vi "Auto.vi"() -> ()   [LabVIEW 2018]
uses:
  Controls/READ CAN CLUSTER.ctl
  CAN_States.ctl
  Controls/FEV_DBC CLUSTER.ctl
  Controls/DBC CLUSTER.ctl
  Controls/CLUSTER.ctl
  CAN Write Data/Application/Common VIs/Read File Data.ctl
  Conf/FGV States.ctl
  cc4f6fa3-47e0-4703-a92c-c7cffe72e988.vi
panel:
  in  "SEND DATA":bool
  in  "TRIGGER":bool
  in  "READ DATA":bool
  in  "exit":bool
  in  "error in (no error)":errorcluster
  out "error out":errorcluster
  in  "WRITE DATA":T1[](array[typedef])
  out "READ DATA":T1[](array[typedef])
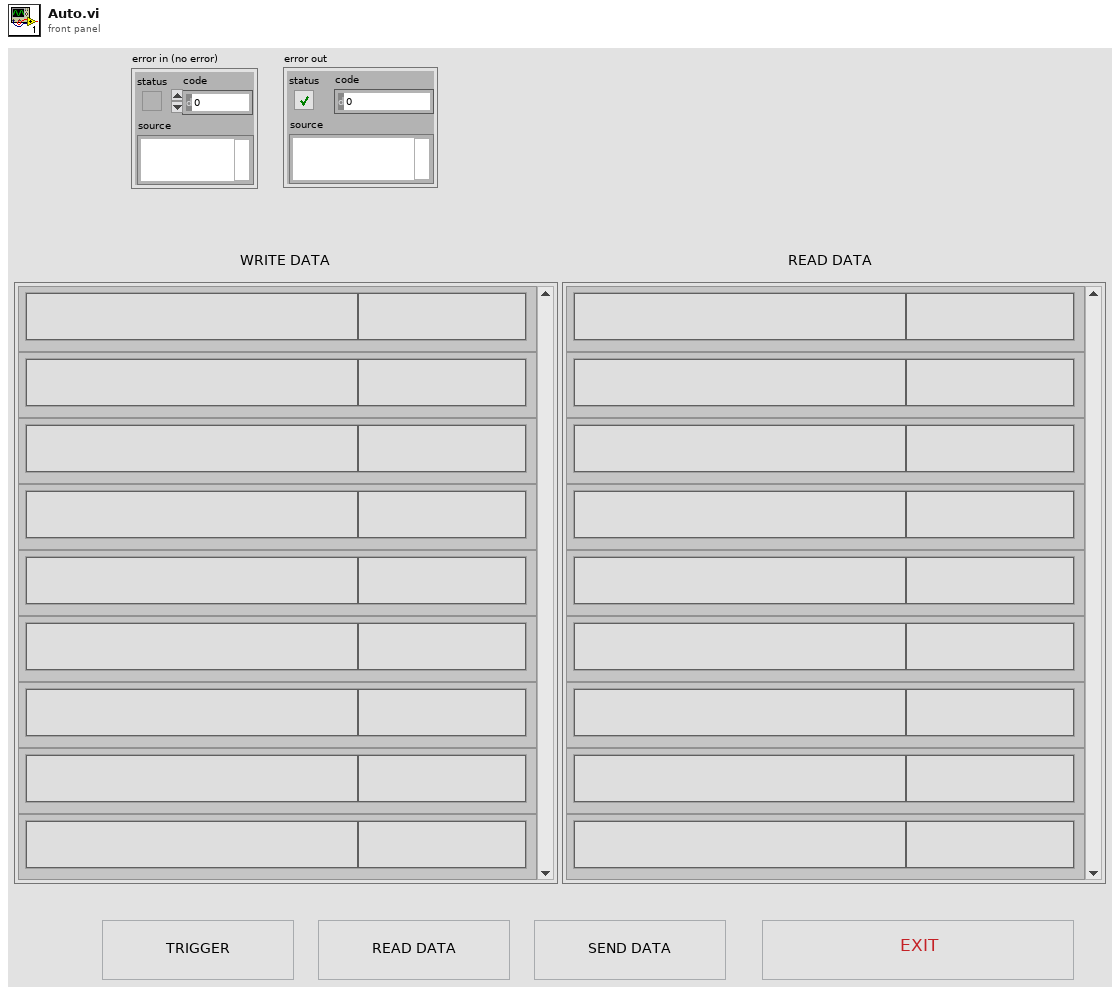
[diagram p1: front panel]
types:
  T1 = typedef "READ CAN CLUSTER.ctl" = cluster{"FUNCTION":string, "DATA":string}
  T2 = typedef "CAN_States.ctl" = enum16{"INT", "NO EVENT", "READ DATA", "WRITE DATA", "EXIT"}
  T3 = typedef "FGV States.ctl" = enum16{"OPEN", "READ", "CLOSE", "WRITE"}
  T4 = typedef "Read File Data.ctl" = enum16{"Get Data", "Set Data"}
  T5 = typedef "CLUSTER.ctl" = cluster{"FUNCTION":string, "READ":bool, "WRITE":bool}
  T6 = typedef "FEV_DBC CLUSTER.ctl" = cluster{"FUNCTION":T7, "DYNO FUNCTION":string}
  T7 = typedef "DBC CLUSTER.ctl" = string
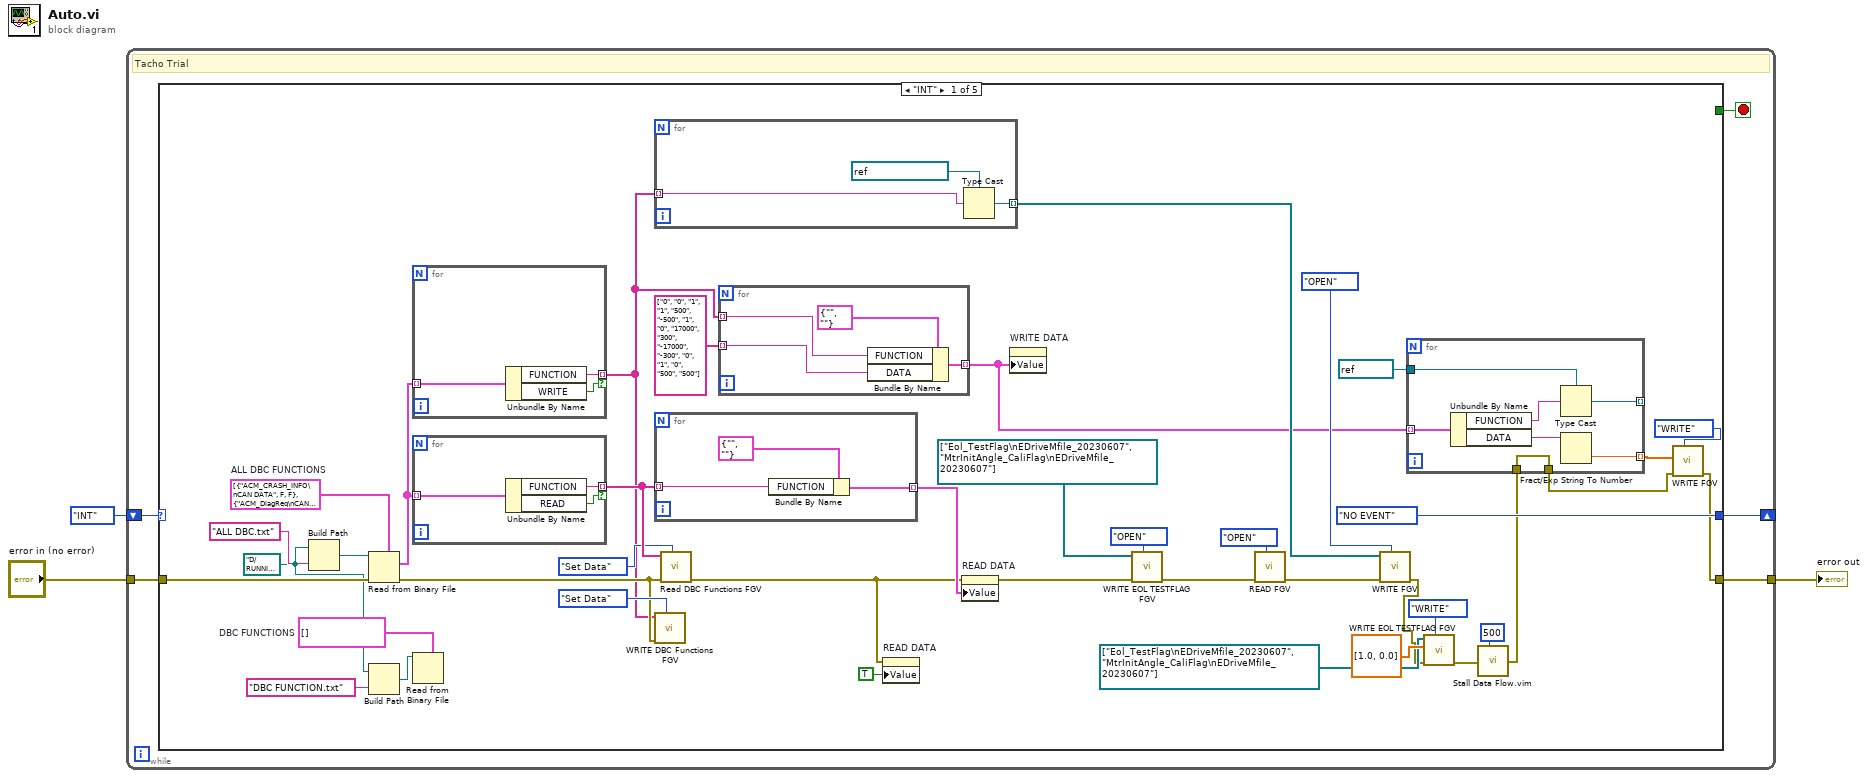
[diagram p0: block diagram]
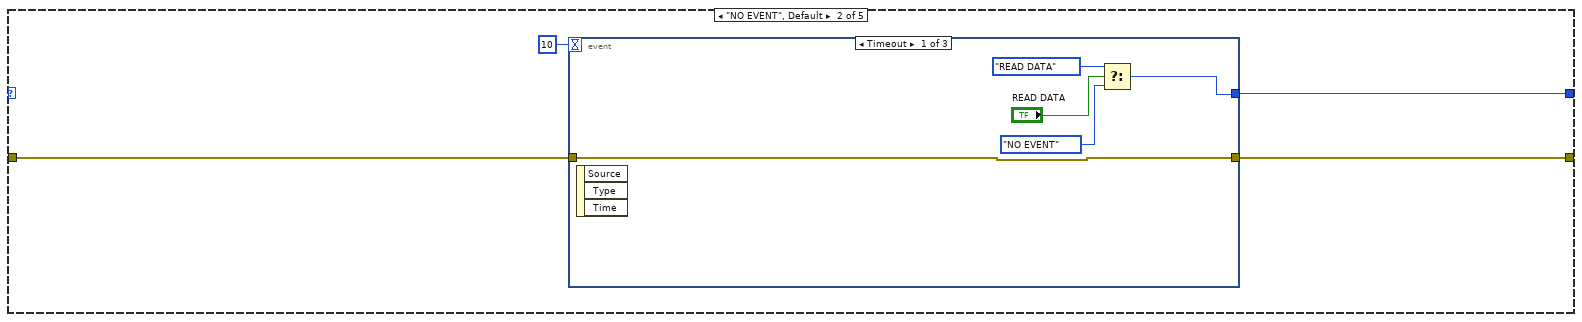
[diagram p2: hidden frame]
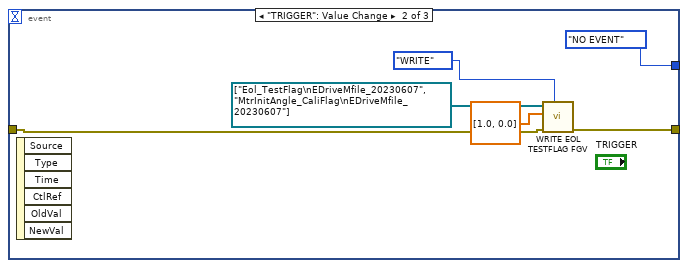
[diagram p3: hidden frame]
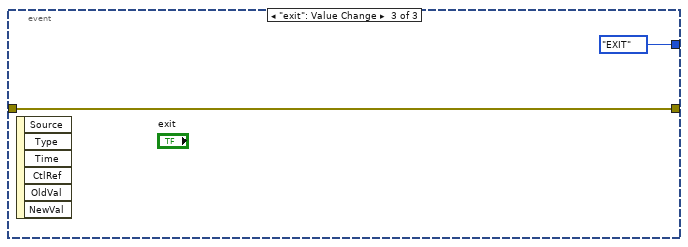
[diagram p4: hidden frame]
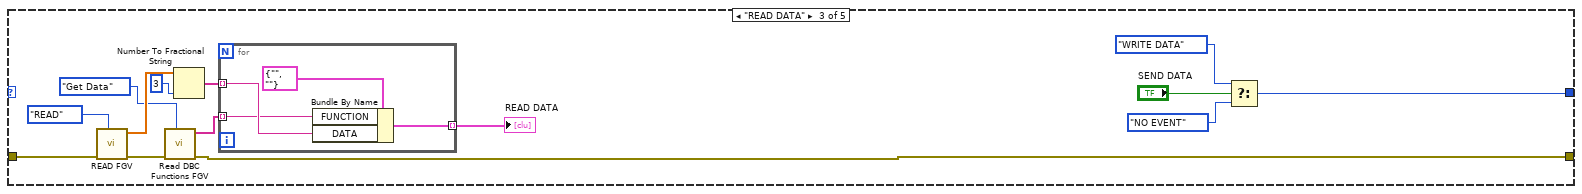
[diagram p5: hidden frame]
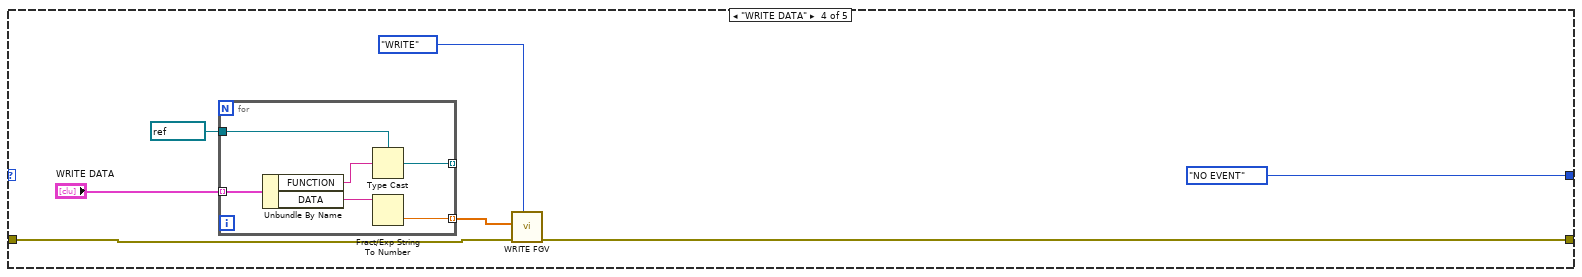
[diagram p6: hidden frame]
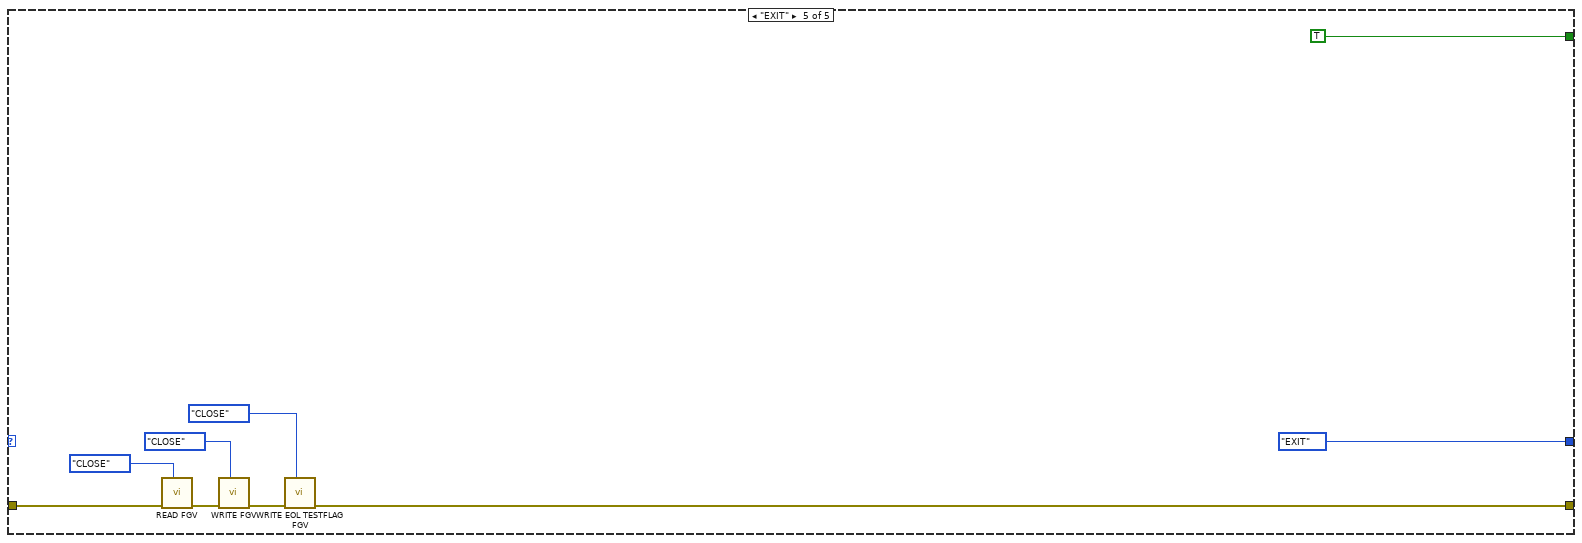
[diagram p7: hidden frame]
diagram:
  n1 = while {
    shift-right: [w7] -> _
    shift-left: CAN_States."INT" -> [w8]
    tunnel: [w6] -> w2
    tunnel: "error in (no error)" -> [w5]
    stop <- w4 stop-if-true
    # "Tacho Trial"
    n2 = case shown="\"INT\"" w8 {
      tunnel: [CAN_States."NO EVENT" w74 w89 CAN_States."NO EVENT" CAN_States."EXIT"] -> w7
      tunnel: [w12 w73 w93 w107 w120] -> w6
      tunnel: w5 -> [w37 w72 w95 w108 w125]
      tunnel: [_ _ _ _ TRUE] -> w4
      frame "INT" {
        w34 = path "D:/RUNNING PROJECT/FEV/#0253/9. Softcode/Source Code/Data/Models/TACO" ("base path")
        w41 = T5[] [{"FUNCTION"="ACM_CRASH_INFO\nCAN DATA", "READ"=FALSE, "WRITE"=FALSE}, {"FUNCTION"="ACM_DiagReq\nCAN DATA", "READ"=FALSE, "WRITE"=FALSE}, {"FUNCTION"="ACM_DiagResp\nCAN DATA", "READ"=FALSE, "WRITE"=FALSE}, {"FUNCTION"="ACM_OCCUPANT_STATUS\nCAN DATA", "READ"=FALSE, "WRITE"=FALSE}, {"FUNCTION"="ACM_WarnMsg\nCAN DATA", "READ"=FALSE, "WRITE"=FALSE}, {"FUNCTION"="ADAS_AEB\nCAN DATA", "READ"=FALSE, "WRITE"=FALSE}, {"FUNCTION"="ADAS_AHB_DOW\nCAN DATA", "READ"=FALSE, "WRITE"=FALSE}, {"FUNCTION"="ADAS_APA_SLOT1INFO1\nCAN DATA", "READ"=FALSE, "WRITE"=FALSE}, {"FUNCTION"="ADAS_APA_SLOT1INFO2\nCAN DATA", "READ"=FALSE, "WRITE"=FALSE}, {"FUNCTION"="ADAS_APA_SLOT1INFO3\nCAN DATA", "READ"=FALSE, "WRITE"=FALSE}, {"FUNCTION"="ADAS_APA_SLOT2INFO1\nCAN DATA", "READ"=FALSE, "WRITE"=FALSE}, {"FUNCTION"="ADAS_APA_SLOT2INFO2\nCAN DATA", "READ"=FALSE, "WRITE"=FALSE}, {"FUNCTION"="ADAS_APA_SLOT2INFO3\nCAN DATA", "READ"=FALSE, "WRITE"=FALSE}, {"FUNCTION"="ADAS_APA_SLOT3INFO1\nCAN DATA", "READ"=FALSE, "WRITE"=FALSE}, {"FUNCTION"="ADAS_APA_SLOT3INFO2\nCAN DATA", "READ"=FALSE, "WRITE"=FALSE}, {"FUNCTION"="ADAS_APA_SLOT3INFO3\nCAN DATA", "READ"=FALSE, "WRITE"=FALSE}, {"FUNCTION"="ADAS_APA_SLOT4INFO1\nCAN DATA", "READ"=FALSE, "WRITE"=FALSE}, {"FUNCTION"="ADAS_APA_SLOT4INFO2\nCAN DATA", "READ"=FALSE, "WRITE"=FALSE}, {"FUNCTION"="ADAS_APA_SLOT4INFO3\nCAN DATA", "READ"=FALSE, "WRITE"=FALSE}, {"FUNCTION"="ADAS_APA_SLOT5INFO1\nCAN DATA", "READ"=FALSE, "WRITE"=FALSE}, {"FUNCTION"="ADAS_APA_SLOT5INFO2\nCAN DATA", "READ"=FALSE, "WRITE"=FALSE}, {"FUNCTION"="ADAS_APA_SLOT5INFO3\nCAN DATA", "READ"=FALSE, "WRITE"=FALSE}, {"FUNCTION"="ADAS_APA_SLOT6INFO1\nCAN DATA", "READ"=FALSE, "WRITE"=FALSE}, {"FUNCTION"="ADAS_APA_SLOT6INFO2\nCAN DATA", "READ"=FALSE, "WRITE"=FALSE}, {"FUNCTION"="ADAS_APA_SLOT6INFO3\nCAN DATA", "READ"=FALSE, "WRITE"=FALSE}, {"FUNCTION"="ADAS_AVM_Sts\nCAN DATA", "READ"=FALSE, "WRITE"=FALSE}, {"FUNCTION"="ADAS_BSD\nCAN DATA", "READ"=FALSE, "WRITE"=FALSE}, {"FUNCTION"="ADAS_CMP_ACC\nCAN DATA", "READ"=FALSE, "WRITE"=FALSE}, {"FUNCTION"="ADAS_CMP_CHECK\nCAN DATA", "READ"=FALSE, "WRITE"=FALSE}, {"FUNCTION"="ADAS_CMP_MHU\nCAN DATA", "READ"=FALSE, "WRITE"=FALSE}, {"FUNCTION"="ADAS_DMS_STATUS\nCAN DATA", "READ"=FALSE, "WRITE"=FALSE}, {"FUNCTION"="ADAS_DiagReq\nCAN DATA", "READ"=FALSE, "WRITE"=FALSE}, {"FUNCTION"="ADAS_DiagResp\nCAN DATA", "READ"=FALSE, "WRITE"=FALSE}, {"FUNCTION"="ADAS_ELK\nCAN DATA", "READ"=FALSE, "WRITE"=FALSE}, {"FUNCTION"="ADAS_FCW_RCTA\nCAN DATA", "READ"=FALSE, "WRITE"=FALSE}, {"FUNCTION"="ADAS_Immo_MHU\nCAN DATA", "READ"=FALSE, "WRITE"=FALSE}, {"FUNCTION"="ADAS_LDW_LKA\nCAN DATA", "READ"=FALSE, "WRITE"=FALSE}, {"FUNCTION"="ADAS_NM\nCAN DATA", "READ"=FALSE, "WRITE"=FALSE}, {"FUNCTION"="ADAS_PA\nCAN DATA", "READ"=FALSE, "WRITE"=FALSE}, {"FUNCTION"="ADAS_RP_Sts\nCAN DATA", "READ"=FALSE, "WRITE"=FALSE}, {"FUNCTION"="ADAS_Speed_Display\nCAN DATA", "READ"=FALSE, "WRITE"=FALSE}, {"FUNCTION"="ADAS_TSR_STATUS\nCAN DATA", "READ"=FALSE, "WRITE"=FALSE}, {"FUNCTION"="ADAS_WarnMsg\nCAN DATA", "READ"=FALSE, "WRITE"=FALSE}, {"FUNCTION"="AMP_DiagReq\nCAN DATA", "READ"=FALSE, "WRITE"=FALSE}, {"FUNCTION"="AMP_DiagResp\nCAN DATA", "READ"=FALSE, "WRITE"=FALSE}, {"FUNCTION"="AMP_MHUEQType\nCAN DATA", "READ"=FALSE, "WRITE"=FALSE}, {"FUNCTION"="AMP_MHU_Ann1_ModeSET\nCAN DATA", "READ"=FALSE, "WRITE"=FALSE}, {"FUNCTION"="AMP_MHU_Ann1_PromptsSET\nCAN DATA", "READ"=FALSE, "WRITE"=FALSE}, {"FUNCTION"="AMP_MHU_Ann2_SpeakerSET\nCAN DATA", "READ"=FALSE, "WRITE"=FALSE}, {"FUNCTION"="AMP_MHU_SET\nCAN DATA", "READ"=FALSE, "WRITE"=FALSE}, {"FUNCTION"="AMP_NM\nCAN DATA", "READ"=FALSE, "WRITE"=FALSE}, {"FUNCTION"="AMP_rDiagReq\nCAN DATA", "READ"=FALSE, "WRITE"=FALSE}, {"FUNCTION"="AMP_rDiagResp\nCAN DATA", "READ"=FALSE, "WRITE"=FALSE}, {"FUNCTION"="APA_FEEDBACK_MHU\nCAN DATA", "READ"=FALSE, "WRITE"=FALSE}, {"FUNCTION"="APA_SENSOR\nCAN DATA", "READ"=FALSE, "WRITE"=FALSE}, {"FUNCTION"="APM_DiagReq\nCAN DATA", "READ"=FALSE, "WRITE"=FALSE}, {"FUNCTION"="APM_DiagResp\nCAN DATA", "READ"=FALSE, "WRITE"=FALSE}, {"FUNCTION"="APM_WINDOW_POS\nCAN DATA", "READ"=FALSE, "WRITE"=FALSE}, {"FUNCTION"="APM_WarnMsg\nCAN DATA", "READ"=FALSE, "WRITE"=FALSE}, {"FUNCTION"="ASU_DiagReq\nCAN DATA", "READ"=FALSE, "WRITE"=FALSE}, {"FUNCTION"="ASU_DiagResp\nCAN DATA", "READ"=FALSE, "WRITE"=FALSE}, {"FUNCTION"="AVAS_DiagReq\nCAN DATA", "READ"=FALSE, "WRITE"=FALSE}, {"FUNCTION"="AVAS_DiagResp\nCAN DATA", "READ"=FALSE, "WRITE"=FALSE}, {"FUNCTION"="AVAS_STATUS\nCAN DATA", "READ"=FALSE, "WRITE"=FALSE}, {"FUNCTION"="BCM_ALM_warning\nCAN DATA", "READ"=FALSE, "WRITE"=FALSE}, {"FUNCTION"="BCM_BPM_DiagReq\nCAN DATA", "READ"=FALSE, "WRITE"=FALSE}, {"FUNCTION"="BCM_BPM_DiagResp\nCAN DATA", "READ"=FALSE, "WRITE"=FALSE}, {"FUNCTION"="BCM_CLAMP_STAT\nCAN DATA", "READ"=FALSE, "WRITE"=FALSE}, {"FUNCTION"="BCM_Comfort_Confirm_sts\nCAN DATA", "READ"=FALSE, "WRITE"=FALSE}, {"FUNCTION"="BCM_DiagReq\nCAN DATA", "READ"=FALSE, "WRITE"=FALSE}, {"FUNCTION"="BCM_DiagResp\nCAN DATA", "READ"=FALSE, "WRITE"=FALSE}, {"FUNCTION"="BCM_ENERGY_MANAGEMENT\nCAN DATA", "READ"=FALSE, "WRITE"=FALSE}, {"FUNCTION"="BCM_ENTRY_CONTROL\nCAN DATA", "READ"=FALSE, "WRITE"=FALSE}, {"FUNCTION"="BCM_FKS_STATUS\nCAN DATA", "READ"=FALSE, "WRITE"=FALSE}, {"FUNCTION"="BCM_LIGHT\nCAN DATA", "READ"=FALSE, "WRITE"=FALSE}, {"FUNCTION"="BCM_LOGICAL_CLAMP\nCAN DATA", "READ"=FALSE, "WRITE"=FALSE}, {"FUNCTION"="BCM_Mirror_Confirm_sts\nCAN DATA", "READ"=FALSE, "WRITE"=FALSE}, {"FUNCTION"="BCM_ODO\nCAN DATA", "READ"=FALSE, "WRITE"=FALSE}, {"FUNCTION"="BCM_RainLightSnr\nCAN DATA", "READ"=FALSE, "WRITE"=FALSE}, {"FUNCTION"="BCM_SCM_LIN_Info\nCAN DATA", "READ"=FALSE, "WRITE"=FALSE}, {"FUNCTION"="BCM_STAT_CENTRAL_LOCK\nCAN DATA", "READ"=FALSE, "WRITE"=FALSE}, {"FUNCTION"="BCM_STAT_DOOR_FLAP\nCAN DATA", "READ"=FALSE, "WRITE"=FALSE}, {"FUNCTION"="BCM_SunroofSts\nCAN DATA", "READ"=FALSE, "WRITE"=FALSE}, {"FUNCTION"="BCM_SunshadeSts\nCAN DATA", "READ"=FALSE, "WRITE"=FALSE}, {"FUNCTION"="BCM_SwitchSts\nCAN DATA", "READ"=FALSE, "WRITE"=FALSE}, {"FUNCTION"="BCM_TERMINAL\nCAN DATA", "READ"=FALSE, "WRITE"=FALSE}, {"FUNCTION"="BCM_VEHICLE_IDENT_NUMBER\nCAN DATA", "READ"=FALSE, "WRITE"=FALSE}, {"FUNCTION"="BCM_VOLTAGE\nCAN DATA", "READ"=FALSE, "WRITE"=FALSE}, {"FUNCTION"="BCM_WarnMsg\nCAN DATA", "READ"=FALSE, "WRITE"=FALSE}, {"FUNCTION"="BMS_CellTemp\nCAN DATA", "READ"=FALSE, "WRITE"=FALSE}, {"FUNCTION"="BMS_ChgParamReq\nCAN DATA", "READ"=FALSE, "WRITE"=FALSE}, {"FUNCTION"="BMS_CurMeas\nCAN DATA", "READ"=FALSE, "WRITE"=FALSE}, {"FUNCTION"="BMS_DiagReq\nCAN DATA", "READ"=FALSE, "WRITE"=FALSE}, {"FUNCTION"="BMS_DiagResp\nCAN DATA", "READ"=FALSE, "WRITE"=FALSE}, {"FUNCTION"="BMS_HVMeas1\nCAN DATA", "READ"=FALSE, "WRITE"=FALSE}, {"FUNCTION"="BMS_Sts\nCAN DATA", "READ"=FALSE, "WRITE"=FALSE}, {"FUNCTION"="BMS_WarnMsg\nCAN DATA", "READ"=FALSE, "WRITE"=FALSE}, {"FUNCTION"="CCUF_DiagReq\nCAN DATA", "READ"=FALSE, "WRITE"=FALSE}, {"FUNCTION"="CCUF_DiagResp\nCAN DATA", "READ"=FALSE, "WRITE"=FALSE}, {"FUNCTION"="CCUR_DiagReq\nCAN DATA", "READ"=FALSE, "WRITE"=FALSE}, {"FUNCTION"="CCUR_DiagResp\nCAN DATA", "READ"=FALSE, "WRITE"=FALSE}, {"FUNCTION"="CCU_STATUS\nCAN DATA", "READ"=FALSE, "WRITE"=FALSE}, {"FUNCTION"="CCU_TEMP_PRESSURE\nCAN DATA", "READ"=FALSE, "WRITE"=FALSE}, {"FUNCTION"="CCU_WarnMsg\nCAN DATA", "READ"=FALSE, "WRITE"=FALSE}, {"FUNCTION"="CPD_DiagReq\nCAN DATA", "READ"=FALSE, "WRITE"=FALSE}, {"FUNCTION"="CPD_DiagResp\nCAN DATA", "READ"=FALSE, "WRITE"=FALSE}, {"FUNCTION"="CPD_NM\nCAN DATA", "READ"=FALSE, "WRITE"=FALSE}, {"FUNCTION"="CPD_OUTPUT\nCAN DATA", "READ"=FALSE, "WRITE"=FALSE}, {"FUNCTION"="CPD_WarnMsg\nCAN DATA", "READ"=FALSE, "WRITE"=FALSE}, {"FUNCTION"="CPD_rDiagReq\nCAN DATA", "READ"=FALSE, "WRITE"=FALSE}, {"FUNCTION"="CPD_rDiagResp\nCAN DATA", "READ"=FALSE, "WRITE"=FALSE}, {"FUNCTION"="Camera_Lane\nCAN DATA", "READ"=FALSE, "WRITE"=FALSE}, {"FUNCTION"="Camera_Object01\nCAN DATA", "READ"=FALSE, "WRITE"=FALSE}, {"FUNCTION"="Camera_Object02\nCAN DATA", "READ"=FALSE, "WRITE"=FALSE}, {"FUNCTION"="Camera_Object03\nCAN DATA", "READ"=FALSE, "WRITE"=FALSE}, {"FUNCTION"="Camera_Object04\nCAN DATA", "READ"=FALSE, "WRITE"=FALSE}, {"FUNCTION"="Camera_Object05\nCAN DATA", "READ"=FALSE, "WRITE"=FALSE}, {"FUNCTION"="Camera_Object06\nCAN DATA", "READ"=FALSE, "WRITE"=FALSE}, {"FUNCTION"="Camera_leftlane\nCAN DATA", "READ"=FALSE, "WRITE"=FALSE}, {"FUNCTION"="Camera_rightlane\nCAN DATA", "READ"=FALSE, "WRITE"=FALSE}, {"FUNCTION"="DCM_APM_DiagReq\nCAN DATA", "READ"=FALSE, "WRITE"=FALSE}, {"FUNCTION"="DCM_APM_DiagResp\nCAN DATA", "READ"=FALSE, "WRITE"=FALSE}, {"FUNCTION"="DIAG_Req_All_CAN\nCAN DATA", "READ"=FALSE, "WRITE"=FALSE}, {"FUNCTION"="DIAG_Req_All_Ecu\nCAN DATA", "READ"=FALSE, "WRITE"=FALSE}, {"FUNCTION"="DIAG_Req_Info\nCAN DATA", "READ"=FALSE, "WRITE"=FALSE}, {"FUNCTION"="DMS_Status\nCAN DATA", "READ"=FALSE, "WRITE"=FALSE}, {"FUNCTION"="Diag_Request_ECU\nCAN DATA", "READ"=FALSE, "WRITE"=FALSE}, {"FUNCTION"="EASC_Confirm_sts\nCAN DATA", "READ"=FALSE, "WRITE"=FALSE}, {"FUNCTION"="EASC_DiagReq\nCAN DATA", "READ"=FALSE, "WRITE"=FALSE}, {"FUNCTION"="EASC_DiagResp\nCAN DATA", "READ"=FALSE, "WRITE"=FALSE}, {"FUNCTION"="EASC_NM\nCAN DATA", "READ"=FALSE, "WRITE"=FALSE}, {"FUNCTION"="EASC_WarnMsg\nCAN DATA", "READ"=FALSE, "WRITE"=FALSE}, {"FUNCTION"="EASC_rDiagReq\nCAN DATA", "READ"=FALSE, "WRITE"=FALSE}, {"FUNCTION"="EASC_rDiagResp\nCAN DATA", "READ"=FALSE, "WRITE"=FALSE}, {"FUNCTION"="EDS_F_DiagReq\nCAN DATA", "READ"=FALSE, "WRITE"=FALSE}, {"FUNCTION"="EDS_F_DiagResp\nCAN DATA", "READ"=FALSE, "WRITE"=FALSE}, {"FUNCTION"="EDS_F_WarnMsg\nCAN DATA", "READ"=FALSE, "WRITE"=FALSE}, {"FUNCTION"="EDS_OutPut_FR\nCAN DATA", "READ"=FALSE, "WRITE"=FALSE}, {"FUNCTION"="EDS_OutPut_RR\nCAN DATA", "READ"=FALSE, "WRITE"=FALSE}, {"FUNCTION"="EDS_R_DiagReq\nCAN DATA", "READ"=FALSE, "WRITE"=FALSE}, {"FUNCTION"="EDS_R_DiagResp\nCAN DATA", "READ"=FALSE, "WRITE"=FALSE}, {"FUNCTION"="EDS_R_WarnMsg\nCAN DATA", "READ"=FALSE, "WRITE"=FALSE}, {"FUNCTION"="EPS2_DiagReq\nCAN DATA", "READ"=FALSE, "WRITE"=FALSE}, {"FUNCTION"="EPS2_DiagResp\nCAN DATA", "READ"=FALSE, "WRITE"=FALSE}, {"FUNCTION"="EPS_DiagReq\nCAN DATA", "READ"=FALSE, "WRITE"=FALSE}, {"FUNCTION"="EPS_DiagResp\nCAN DATA", "READ"=FALSE, "WRITE"=FALSE}, {"FUNCTION"="EPS_WarnMsg\nCAN DATA", "READ"=FALSE, "WRITE"=FALSE}, {"FUNCTION"="ETG_DiagReq\nCAN DATA", "READ"=FALSE, "WRITE"=FALSE}, {"FUNCTION"="ETG_DiagResp\nCAN DATA", "READ"=FALSE, "WRITE"=FALSE}, {"FUNCTION"="ETG_STATUS\nCAN DATA", "READ"=FALSE, "WRITE"=FALSE}, {"FUNCTION"="ETG_WarnMsg\nCAN DATA", "READ"=FALSE, "WRITE"=FALSE}, {"FUNCTION"="GS_DiagReq\nCAN DATA", "READ"=FALSE, "WRITE"=FALSE}, {"FUNCTION"="GS_DiagResp\nCAN DATA", "READ"=FALSE, "WRITE"=FALSE}, {"FUNCTION"="GS_WarnMsg\nCAN DATA", "READ"=FALSE, "WRITE"=FALSE}, {"FUNCTION"="GW_BCM_Immo_MHU_Byte\nCAN DATA", "READ"=FALSE, "WRITE"=FALSE}, {"FUNCTION"="GW_BCM_RemoteCtrlSts\nCAN DATA", "READ"=FALSE, "WRITE"=FALSE}, {"FUNCTION"="HOD_Heating\nCAN DATA", "READ"=FALSE, "WRITE"=FALSE}, {"FUNCTION"="HOD_Heating_FDBK\nCAN DATA", "READ"=FALSE, "WRITE"=FALSE}, {"FUNCTION"="HUD_DiagReq\nCAN DATA", "READ"=FALSE, "WRITE"=FALSE}, {"FUNCTION"="HUD_DiagResp\nCAN DATA", "READ"=FALSE, "WRITE"=FALSE}, {"FUNCTION"="HUD_ECU_Status\nCAN DATA", "READ"=FALSE, "WRITE"=FALSE}, {"FUNCTION"="HUD_NM\nCAN DATA", "READ"=FALSE, "WRITE"=FALSE}, {"FUNCTION"="HUD_State\nCAN DATA", "READ"=FALSE, "WRITE"=FALSE}, {"FUNCTION"="HUD_WarnMsg\nCAN DATA", "READ"=FALSE, "WRITE"=FALSE}, {"FUNCTION"="HUD_rDiagReq\nCAN DATA", "READ"=FALSE, "WRITE"=FALSE}, {"FUNCTION"="HUD_rDiagResp\nCAN DATA", "READ"=FALSE, "WRITE"=FALSE}, {"FUNCTION"="IC_BORD_COMP_TRIP_A\nCAN DATA", "READ"=FALSE, "WRITE"=FALSE}, {"FUNCTION"="IC_BORD_COMP_TRIP_Auto\nCAN DATA", "READ"=FALSE, "WRITE"=FALSE}, {"FUNCTION"="IC_BORD_COMP_TRIP_B\nCAN DATA", "READ"=FALSE, "WRITE"=FALSE}, {"FUNCTION"="IC_MILEAGE\nCAN DATA", "READ"=FALSE, "WRITE"=FALSE}, {"FUNCTION"="IC_ODO\nCAN DATA", "READ"=FALSE, "WRITE"=FALSE}, {"FUNCTION"="IC_RELATIVIME\nCAN DATA", "READ"=FALSE, "WRITE"=FALSE}, {"FUNCTION"="IC_SENSOR\nCAN DATA", "READ"=FALSE, "WRITE"=FALSE}, {"FUNCTION"="IC_STAT_AIRBAG\nCAN DATA", "READ"=FALSE, "WRITE"=FALSE}, {"FUNCTION"="IDB_ACC_LONG_LAT_YAW\nCAN DATA", "READ"=FALSE, "WRITE"=FALSE}, {"FUNCTION"="IDB_DiagReq\nCAN DATA", "READ"=FALSE, "WRITE"=FALSE}, {"FUNCTION"="IDB_DiagResp\nCAN DATA", "READ"=FALSE, "WRITE"=FALSE}, {"FUNCTION"="IDB_EPB_STATUS\nCAN DATA", "READ"=FALSE, "WRITE"=FALSE}, {"FUNCTION"="IDB_FUNCTION\nCAN DATA", "READ"=FALSE, "WRITE"=FALSE}, {"FUNCTION"="IDB_MILEAGE\nCAN DATA", "READ"=FALSE, "WRITE"=FALSE}, {"FUNCTION"="IDB_STATUS\nCAN DATA", "READ"=FALSE, "WRITE"=FALSE}, {"FUNCTION"="IDB_V_VEH\nCAN DATA", "READ"=FALSE, "WRITE"=FALSE}, {"FUNCTION"="IDB_WarnMsg\nCAN DATA", "READ"=FALSE, "WRITE"=FALSE}, {"FUNCTION"="LDML_LIGHT\nCAN DATA", "READ"=FALSE, "WRITE"=FALSE}, {"FUNCTION"="LDMR_LIGHT\nCAN DATA", "READ"=FALSE, "WRITE"=FALSE}, {"FUNCTION"="LDM_L_DiagReq\nCAN DATA", "READ"=FALSE, "WRITE"=FALSE}, {"FUNCTION"="LDM_L_DiagResp\nCAN DATA", "READ"=FALSE, "WRITE"=FALSE}, {"FUNCTION"="LDM_R_DiagReq\nCAN DATA", "READ"=FALSE, "WRITE"=FALSE}, {"FUNCTION"="LDM_R_DiagResp\nCAN DATA", "READ"=FALSE, "WRITE"=FALSE}, {"FUNCTION"="MFS_Control_Button\nCAN DATA", "READ"=FALSE, "WRITE"=FALSE}, {"FUNCTION"="MHU_ADAS_RP_Ctrl\nCAN DATA", "READ"=FALSE, "WRITE"=FALSE}, {"FUNCTION"="MHU_ADAS_RSSI\nCAN DATA", "READ"=FALSE, "WRITE"=FALSE}, {"FUNCTION"="MHU_ADAS_req\nCAN DATA", "READ"=FALSE, "WRITE"=FALSE}, {"FUNCTION"="MHU_AMP_Ann1_ModeSET\nCAN DATA", "READ"=FALSE, "WRITE"=FALSE}, {"FUNCTION"="MHU_AMP_Ann1_PromptsSET\nCAN DATA", "READ"=FALSE, "WRITE"=FALSE}, {"FUNCTION"="MHU_AMP_Ann2_SpeakerSET\nCAN DATA", "READ"=FALSE, "WRITE"=FALSE}, {"FUNCTION"="MHU_AmpEQType\nCAN DATA", "READ"=FALSE, "WRITE"=FALSE}, {"FUNCTION"="MHU_AmpSET\nCAN DATA", "READ"=FALSE, "WRITE"=FALSE}, {"FUNCTION"="MHU_Auth_Immo\nCAN DATA", "READ"=FALSE, "WRITE"=FALSE}, {"FUNCTION"="MHU_Auth_Immo_ADAS\nCAN DATA", "READ"=FALSE, "WRITE"=FALSE}, {"FUNCTION"="MHU_Avas_Setting\nCAN DATA", "READ"=FALSE, "WRITE"=FALSE}, {"FUNCTION"="MHU_BCM_Color_Req\nCAN DATA", "READ"=FALSE, "WRITE"=FALSE}, {"FUNCTION"="MHU_BCM_DoorsCtrl\nCAN DATA", "READ"=FALSE, "WRITE"=FALSE}, {"FUNCTION"="MHU_BCM_HornLightControl\nCAN DATA", "READ"=FALSE, "WRITE"=FALSE}, {"FUNCTION"="MHU_BCM_IntensityTiming_Req\nCAN DATA", "READ"=FALSE, "WRITE"=FALSE}, {"FUNCTION"="MHU_BCM_RemoteClampCtrl\nCAN DATA", "READ"=FALSE, "WRITE"=FALSE}, {"FUNCTION"="MHU_CCUF_ClimateSetting\nCAN DATA", "READ"=FALSE, "WRITE"=FALSE}, {"FUNCTION"="MHU_CCUR_ClimateSetting\nCAN DATA", "READ"=FALSE, "WRITE"=FALSE}, {"FUNCTION"="MHU_CPD_Confirm\nCAN DATA", "READ"=FALSE, "WRITE"=FALSE}, {"FUNCTION"="MHU_CarMode_Switch\nCAN DATA", "READ"=FALSE, "WRITE"=FALSE}, {"FUNCTION"="MHU_ComfortSetting\nCAN DATA", "READ"=FALSE, "WRITE"=FALSE}, {"FUNCTION"="MHU_DATE_TIME\nCAN DATA", "READ"=FALSE, "WRITE"=FALSE}, {"FUNCTION"="MHU_DIGIT_SPEED\nCAN DATA", "READ"=FALSE, "WRITE"=FALSE}, {"FUNCTION"="MHU_DMS_STATUS\nCAN DATA", "READ"=FALSE, "WRITE"=FALSE}, {"FUNCTION"="MHU_DRIVER_INFO\nCAN DATA", "READ"=FALSE, "WRITE"=FALSE}, {"FUNCTION"="MHU_DiagReq\nCAN DATA", "READ"=FALSE, "WRITE"=FALSE}, {"FUNCTION"="MHU_DiagResp\nCAN DATA", "READ"=FALSE, "WRITE"=FALSE}, {"FUNCTION"="MHU_DoorSetting\nCAN DATA", "READ"=FALSE, "WRITE"=FALSE}, {"FUNCTION"="MHU_EvSetting\nCAN DATA", "READ"=FALSE, "WRITE"=FALSE}, {"FUNCTION"="MHU_FEEDBACK_APA\nCAN DATA", "READ"=FALSE, "WRITE"=FALSE}, {"FUNCTION"="MHU_FOTA_ReqAll\nCAN DATA", "READ"=FALSE, "WRITE"=FALSE}, {"FUNCTION"="MHU_FOTA_STATUS\nCAN DATA", "READ"=FALSE, "WRITE"=FALSE}, {"FUNCTION"="MHU_HEADLAMP_CTL\nCAN DATA", "READ"=FALSE, "WRITE"=FALSE}, {"FUNCTION"="MHU_HUD_BASE\nCAN DATA", "READ"=FALSE, "WRITE"=FALSE}, {"FUNCTION"="MHU_HUD_Info_1\nCAN DATA", "READ"=FALSE, "WRITE"=FALSE}, {"FUNCTION"="MHU_HUD_NAV_DISP\nCAN DATA", "READ"=FALSE, "WRITE"=FALSE}, {"FUNCTION"="MHU_HUD_NAV_GuidanceCont\nCAN DATA", "READ"=FALSE, "WRITE"=FALSE}, {"FUNCTION"="MHU_HudPositionSetting\nCAN DATA", "READ"=FALSE, "WRITE"=FALSE}, {"FUNCTION"="MHU_HudSetting\nCAN DATA", "READ"=FALSE, "WRITE"=FALSE}, {"FUNCTION"="MHU_IDB_Mode_Select\nCAN DATA", "READ"=FALSE, "WRITE"=FALSE}, {"FUNCTION"="MHU_ISA_Speed\nCAN DATA", "READ"=FALSE, "WRITE"=FALSE}, {"FUNCTION"="MHU_LightSetting\nCAN DATA", "READ"=FALSE, "WRITE"=FALSE}, {"FUNCTION"="MHU_MirrorAdjust\nCAN DATA", "READ"=FALSE, "WRITE"=FALSE}, {"FUNCTION"="MHU_NAV_JUNC_INFO\nCAN DATA", "READ"=FALSE, "WRITE"=FALSE}, {"FUNCTION"="MHU_NM\nCAN DATA", "READ"=FALSE, "WRITE"=FALSE}, {"FUNCTION"="MHU_SEAT_CONTROL\nCAN DATA", "READ"=FALSE, "WRITE"=FALSE}, {"FUNCTION"="MHU_STATUS\nCAN DATA", "READ"=FALSE, "WRITE"=FALSE}, {"FUNCTION"="MHU_SeatVentHeat\nCAN DATA", "READ"=FALSE, "WRITE"=FALSE}, {"FUNCTION"="MHU_SteeringAdjust\nCAN DATA", "READ"=FALSE, "WRITE"=FALSE}, {"FUNCTION"="MHU_UserProfile\nCAN DATA", "READ"=FALSE, "WRITE"=FALSE}, {"FUNCTION"="MHU_WindowSetting\nCAN DATA", "READ"=FALSE, "WRITE"=FALSE}, {"FUNCTION"="MRGEN_DiagReq\nCAN DATA", "READ"=FALSE, "WRITE"=FALSE}, {"FUNCTION"="MRGEN_DiagResp\nCAN DATA", "READ"=FALSE, "WRITE"=FALSE}, {"FUNCTION"="OCS_P_DiagReq\nCAN DATA", "READ"=FALSE, "WRITE"=FALSE}, {"FUNCTION"="OCS_P_DiagResp\nCAN DATA", "READ"=FALSE, "WRITE"=FALSE}, {"FUNCTION"="POD_DCDC_DiagReq\nCAN DATA", "READ"=FALSE, "WRITE"=FALSE}, {"FUNCTION"="POD_DCDC_DiagResp\nCAN DATA", "READ"=FALSE, "WRITE"=FALSE}, {"FUNCTION"="POD_GW_Request\nCAN DATA", "READ"=FALSE, "WRITE"=FALSE}, {"FUNCTION"="POD_GW_Response\nCAN DATA", "READ"=FALSE, "WRITE"=FALSE}, {"FUNCTION"="POD_OBC_DiagReq\nCAN DATA", "READ"=FALSE, "WRITE"=FALSE}, {"FUNCTION"="POD_OBC_DiagResp\nCAN DATA", "READ"=FALSE, "WRITE"=FALSE}, {"FUNCTION"="POD_WarnMsg\nCAN DATA", "READ"=FALSE, "WRITE"=FALSE}, {"FUNCTION"="PSM_D_DiagReq\nCAN DATA", "READ"=FALSE, "WRITE"=FALSE}, {"FUNCTION"="PSM_D_DiagResp\nCAN DATA", "READ"=FALSE, "WRITE"=FALSE}, {"FUNCTION"="PSM_D_SEAT_CONTROL\nCAN DATA", "READ"=FALSE, "WRITE"=FALSE}, {"FUNCTION"="PSM_SEAT_POSITION\nCAN DATA", "READ"=FALSE, "WRITE"=FALSE}, {"FUNCTION"="PSM_WarnMsg\nCAN DATA", "READ"=FALSE, "WRITE"=FALSE}, {"FUNCTION"="RCU_DiagReq\nCAN DATA", "READ"=FALSE, "WRITE"=FALSE}, {"FUNCTION"="RCU_DiagResp\nCAN DATA", "READ"=FALSE, "WRITE"=FALSE}, {"FUNCTION"="RCU_WarnMsg\nCAN DATA", "READ"=FALSE, "WRITE"=FALSE}, {"FUNCTION"="SAS_Sensor\nCAN DATA", "READ"=FALSE, "WRITE"=FALSE}, {"FUNCTION"="SCAM_DiagReq\nCAN DATA", "READ"=FALSE, "WRITE"=FALSE}, {"FUNCTION"="SCAM_DiagResp\nCAN DATA", "READ"=FALSE, "WRITE"=FALSE}, {"FUNCTION"="SCM_Raw_Status\nCAN DATA", "READ"=FALSE, "WRITE"=FALSE}, {"FUNCTION"="SHVU_F_Confirm_Sts\nCAN DATA", "READ"=FALSE, "WRITE"=FALSE}, {"FUNCTION"="SHVU_F_DiagReq\nCAN DATA", "READ"=FALSE, "WRITE"=FALSE}, {"FUNCTION"="SHVU_F_DiagResp\nCAN DATA", "READ"=FALSE, "WRITE"=FALSE}, {"FUNCTION"="SHVU_R_Confirm_Sts\nCAN DATA", "READ"=FALSE, "WRITE"=FALSE}, {"FUNCTION"="SHVU_R_DiagReq\nCAN DATA", "READ"=FALSE, "WRITE"=FALSE}, {"FUNCTION"="SHVU_R_DiagResp\nCAN DATA", "READ"=FALSE, "WRITE"=FALSE}, {"FUNCTION"="SRR_FL_DiagReq\nCAN DATA", "READ"=FALSE, "WRITE"=FALSE}, {"FUNCTION"="SRR_FL_DiagResp\nCAN DATA", "READ"=FALSE, "WRITE"=FALSE}, {"FUNCTION"="SRR_FR_DiagReq\nCAN DATA", "READ"=FALSE, "WRITE"=FALSE}, {"FUNCTION"="SRR_FR_DiagResp\nCAN DATA", "READ"=FALSE, "WRITE"=FALSE}, {"FUNCTION"="SRR_RL_DiagReq\nCAN DATA", "READ"=FALSE, "WRITE"=FALSE}, {"FUNCTION"="SRR_RL_DiagResp\nCAN DATA", "READ"=FALSE, "WRITE"=FALSE}, {"FUNCTION"="SRR_RR_DiagReq\nCAN DATA", "READ"=FALSE, "WRITE"=FALSE}, {"FUNCTION"="SRR_RR_DiagResp\nCAN DATA", "READ"=FALSE, "WRITE"=FALSE}, {"FUNCTION"="SeatMassage_Input\nCAN DATA", "READ"=FALSE, "WRITE"=FALSE}, {"FUNCTION"="SeatMassage_Output\nCAN DATA", "READ"=FALSE, "WRITE"=FALSE}, {"FUNCTION"="Sensor_Fault\nCAN DATA", "READ"=FALSE, "WRITE"=FALSE}, {"FUNCTION"="TPMS_TirePressure\nCAN DATA", "READ"=FALSE, "WRITE"=FALSE}, {"FUNCTION"="TRM_DiagReq\nCAN DATA", "READ"=FALSE, "WRITE"=FALSE}, {"FUNCTION"="TRM_DiagResp\nCAN DATA", "READ"=FALSE, "WRITE"=FALSE}, {"FUNCTION"="TRM_WarnMsg\nCAN DATA", "READ"=FALSE, "WRITE"=FALSE}, {"FUNCTION"="VCU_ChargingConnection\nCAN DATA", "READ"=FALSE, "WRITE"=FALSE}, {"FUNCTION"="VCU_DiagReq\nCAN DATA", "READ"=FALSE, "WRITE"=FALSE}, {"FUNCTION"="VCU_DiagResp\nCAN DATA", "READ"=FALSE, "WRITE"=FALSE}, {"FUNCTION"="VCU_HMI_Info\nCAN DATA", "READ"=FALSE, "WRITE"=FALSE}, {"FUNCTION"="VCU_HV_DrvSys_status\nCAN DATA", "READ"=FALSE, "WRITE"=FALSE}, {"FUNCTION"="VCU_HVsystem_status\nCAN DATA", "READ"=FALSE, "WRITE"=FALSE}, {"FUNCTION"="VCU_MHU_info\nCAN DATA", "READ"=FALSE, "WRITE"=FALSE}, {"FUNCTION"="VCU_WarnMsg\nCAN DATA", "READ"=FALSE, "WRITE"=FALSE}, {"FUNCTION"="WLC_Status\nCAN DATA", "READ"=FALSE, "WRITE"=FALSE}, {"FUNCTION"="WLC_Status_2\nCAN DATA", "READ"=FALSE, "WRITE"=FALSE}, {"FUNCTION"="XGW_DiagReq\nCAN DATA", "READ"=FALSE, "WRITE"=FALSE}, {"FUNCTION"="XGW_DiagResp\nCAN DATA", "READ"=FALSE, "WRITE"=FALSE}, {"FUNCTION"="XGW_FOTA_StsConfirm\nCAN DATA", "READ"=FALSE, "WRITE"=FALSE}, {"FUNCTION"="XGW_HCMInfo\nCAN DATA", "READ"=FALSE, "WRITE"=FALSE}, {"FUNCTION"="XGW_Info_Collect\nCAN DATA", "READ"=FALSE, "WRITE"=FALSE}, {"FUNCTION"="XGW_NM\nCAN DATA", "READ"=FALSE, "WRITE"=FALSE}, {"FUNCTION"="XGW_System_Info\nCAN DATA", "READ"=FALSE, "WRITE"=FALSE}, {"FUNCTION"="XGW_WarnMsg\nCAN DATA", "READ"=FALSE, "WRITE"=FALSE}, {"FUNCTION"="YSS_DiagReq\nCAN DATA", "READ"=FALSE, "WRITE"=FALSE}, {"FUNCTION"="YSS_DiagResp\nCAN DATA", "READ"=FALSE, "WRITE"=FALSE}]  # ALL DBC FUNCTIONS
        w42 = T6[] []  # DBC FUNCTIONS
        n3 = Build Path(base path=w34, name or relative path="ALL DBC.txt") -> (appended path=w45:path)
        n4 = Read from Binary File(5:w41, 8:w37, 11:w45) -> (0:w36:errorcluster, 2:w47:T5[])  [unwired: 3 in, 2 out]
        n5 = Build Path(base path=w34, name or relative path="DBC FUNCTION.txt") -> (appended path=w46:path)
        n6 = for {
          tunnel: w47 -> [w68] mode=indexing
          tunnel: [w67] -> w29 mode=indexing if=w66
          n7 = Unbundle By Name(w68) -> ("FUNCTION"=w67:string, "WRITE"=w66:bool)
        }
        n8 = for {
          tunnel: w47 -> [w71] mode=indexing
          tunnel: [w70] -> w48 mode=indexing if=w69
          n9 = Unbundle By Name(w71) -> ("FUNCTION"=w70:string, "READ"=w69:bool)
        }
        n10 = Read from Binary File(5:w42, 11:w46) -> ()  [unwired: 4 in, 4 out]
        n11 = for {
          tunnel: w29 -> [w58] mode=indexing
          tunnel: [w56] -> w28 mode=indexing
          n12 = Type Cast(type=refnum<k21> "EngineOilPrLamp\nTEST" ("XNET Signal"), x=w58) -> (*(type *) &x=w56:refnum<k21>)
        }
        n13 = for {
          tunnel: w48 -> [w64] mode=indexing
          tunnel: [w63] -> w35 mode=indexing
          n14 = Bundle By Name(cluster=T1 {"FUNCTION"="", "DATA"=""} ("FUNCTIONS"), "FUNCTION"=w64) -> (w63:T1)
        }
        n15 = call "WRITE DBC Functions FGV.vi"("Enum"=Read_File_Data."Set Data", "error in (no error)"=w36, "DBC FUNCTIONS IN"=w29) -> ()  [unwired: 7 in, 2 out]
        n16 = call "Read DBC Functions FGV.vi"("Enum"=Read_File_Data."Set Data", "error in (no error)"=w36, "DBC FUNCTIONS IN"=w48) -> ("error out"=w9:errorcluster)  [unwired: 7 in, 1 out]
        n17 = for {
          tunnel: w29 -> [w61] mode=indexing
          tunnel: [w60] -> w11 mode=indexing
          tunnel: string[] ["0", "0", "1", "1", "500", "-500", "1", "0", "17000", "300", "-17000", "-300", "0", "1", "0", "500", "500"] ("Array 2") -> [w59] mode=indexing
          n18 = Bundle By Name(cluster=T1 {"FUNCTION"="", "DATA"=""} ("FUNCTIONS"), "FUNCTION"=w61, "DATA"=w59) -> (w60:T1)
        }
        n19 = property on="READ DATA" class="Bool (strict)"(error in=w9, "Value"=TRUE ("READ DATA")) -> ()  [unwired: 1 in, 2 out]
        n20 = property on="READ DATA" class="Arr (strict)"(error in=w9, "Value"=w35) -> (error out=w26:errorcluster)  [unwired: 1 in, 1 out]
        n21 = property on="WRITE DATA" class="Arr (strict)"("Value"=w11) -> ()  [unwired: 2 in, 2 out]
        n22 = call "WRITE EOL TESTFLAG FGV.vi"("Enum"=FGV_States."OPEN", "error in (no error)"=w26, "signal list"=refnum<k21>[] ["Eol_TestFlag\nEDriveMfile_20230607", "MtrInitAngle_CaliFlag\nEDriveMfile_20230607"]) -> ("error out"=w25:errorcluster)  [unwired: 8 in]
        n23 = call "READ FGV.vi"("Enum"=FGV_States."OPEN", "error in (no error)"=w25) -> ("error out"=w30:errorcluster)  [unwired: 8 in, 1 out]
        n24 = call "WRITE FGV.vi"("Enum"=FGV_States."OPEN", "error in (no error)"=w30, "signal list"=w28) -> ("error out"=w20:errorcluster)  [unwired: 8 in]
        n25 = call "WRITE EOL TESTFLAG FGV.vi"("Enum"=FGV_States."WRITE", "error in (no error)"=w20, "data"=dbl[] [1.0, 0.0], "signal list"=refnum<k21>[] ["Eol_TestFlag\nEDriveMfile_20230607", "MtrInitAngle_CaliFlag\nEDriveMfile_20230607"]) -> ("error out"=w16:errorcluster)  [unwired: 7 in]
        n26 = call "Stall Data Flow.vim"("value in"=w16, "milliseconds to wait"=u32 500) -> ("value out"=w13:errorcluster)  [unwired: 1 out]
        n27 = for {
          tunnel: w11 -> [w55] mode=indexing
          tunnel: [w53] -> w19 mode=indexing
          tunnel: refnum<k21> "EngineOilPrLamp\nTEST" ("XNET Signal") -> [w52]
          tunnel: [w50] -> _ mode=indexing
          tunnel: [w49] -> w14
          tunnel: w13 -> [w49]
          n28 = Unbundle By Name(w55) -> ("FUNCTION"=w51:string, "DATA"=w54:string)
          n29 = Type Cast(type=w52, x=w51) -> (*(type *) &x=w50:refnum<k21>)
          n30 = Fract/Exp String To Number(string=w54) -> (number=w53:dbl)  [unwired: 3 in, 1 out]
        }
        n31 = call "WRITE FGV.vi"("Enum"=FGV_States."WRITE", "error in (no error)"=w14, "data"=w19) -> ("error out"=w12:errorcluster)  [unwired: 8 in]
      }
      frame "NO EVENT", Default {
        n32 = event shown="[0] Timeout" {
          selector: _ -> [_ _ _]
          dyn-events: _ -> [_ _ _]
          timeout: 10 -> [_ _ _]
          tunnel: [w77 CAN_States."NO EVENT" CAN_States."EXIT"] -> w74
          tunnel: [w80 w83 w88] -> w73
          tunnel: w72 -> [w80 w84 w88]
          event Timeout {
            n33 = event-data() -> ()  [unwired: 1 in, 3 out]
            n34 = Select(t=CAN_States."READ DATA", s="READ DATA", f=CAN_States."NO EVENT") -> (s? t:f=w77:T2)
          }
          event "TRIGGER": Value Change {
            n35 = event-data() -> ()  [unwired: 1 in, 6 out]
            n36 = call "WRITE EOL TESTFLAG FGV.vi"("Enum"=FGV_States."WRITE", "error in (no error)"=w84, "data"=dbl[] [1.0, 0.0], "signal list"=refnum<k21>[] ["Eol_TestFlag\nEDriveMfile_20230607", "MtrInitAngle_CaliFlag\nEDriveMfile_20230607"]) -> ("error out"=w83:errorcluster)  [unwired: 7 in]
          }
          event "exit": Value Change {
            n37 = event-data() -> ()  [unwired: 1 in, 6 out]
          }
        }
      }
      frame "READ DATA" {
        n38 = call "READ FGV.vi"("Enum"=FGV_States."READ", "error in (no error)"=w95) -> ("error out"=w94:errorcluster, "data"=w99:dbl[])  [unwired: 8 in]
        n39 = call "Read DBC Functions FGV.vi"("Enum"=Read_File_Data."Get Data", "error in (no error)"=w94) -> ("error out"=w93:errorcluster, "DBC FUNCTIONS OUT"=w100:string[])  [unwired: 8 in]
        n40 = Number To Fractional String(number=w99, precision (6)=i16 3) -> (F-format string=w101:string[])  [unwired: 2 in]
        n41 = for {
          tunnel: w101 -> [w105] mode=indexing
          tunnel: [w104] -> w102 mode=indexing
          tunnel: w100 -> [w103] mode=indexing
          n42 = Bundle By Name(cluster=T1 {"FUNCTION"="", "DATA"=""} ("FUNCTIONS"), "FUNCTION"=w103, "DATA"=w105) -> (w104:T1)
        }
        "READ DATA" <- w102
        n43 = Select(t=CAN_States."WRITE DATA", s="SEND DATA", f=CAN_States."NO EVENT") -> (s? t:f=w89:T2)
      }
      frame "WRITE DATA" {
        n44 = for {
          tunnel: "WRITE DATA" -> [w119] mode=indexing
          tunnel: [w117] -> w112 mode=indexing
          tunnel: refnum<k21> "EngineOilPrLamp\nTEST" ("XNET Signal") -> [w116]
          tunnel: [w114] -> _ mode=indexing
          n45 = Unbundle By Name(w119) -> ("FUNCTION"=w115:string, "DATA"=w118:string)
          n46 = Type Cast(type=w116, x=w115) -> (*(type *) &x=w114:refnum<k21>)
          n47 = Fract/Exp String To Number(string=w118) -> (number=w117:dbl)  [unwired: 3 in, 1 out]
        }
        n48 = call "WRITE FGV.vi"("Enum"=FGV_States."WRITE", "error in (no error)"=w108, "data"=w112) -> ("error out"=w107:errorcluster)  [unwired: 8 in]
      }
      frame "EXIT" {
        n49 = call "READ FGV.vi"("Enum"=FGV_States."CLOSE", "error in (no error)"=w125) -> ("error out"=w123:errorcluster)  [unwired: 8 in, 1 out]
        n50 = call "WRITE FGV.vi"("Enum"=FGV_States."CLOSE", "error in (no error)"=w123) -> ("error out"=w121:errorcluster)  [unwired: 9 in]
        n51 = call "WRITE EOL TESTFLAG FGV.vi"("Enum"=FGV_States."CLOSE", "error in (no error)"=w121) -> ("error out"=w120:errorcluster)  [unwired: 9 in]
      }
    }
  }
  "error out" <- w2
